vi "test_acquire_image.vi"() -> ()   [LabVIEW 2019, in "Picam.lvclass"]
uses:
  Picam.lvclass
  picam32_LabView_SDK/PICam_lib/types/PicamModel.ctl
  picam32_LabView_SDK/PICam_lib/types/PicamRoi.ctl
panel:
  in  "PicamRoi":T1={"x"=0, "width"=1024, "x_binning"=8, "y"=0, "height"=1024, "y_binning"=4}
  out "size(s)":i32[](array[numeric])
  out "ReadoutCount":i64
  out "Image":u16[][](graph)
  out "error out":errorcluster
  in  "PicamModel":T2=715 items=["---PIXIS 100 SERIES---"=1000, "PixisSeries"=0, "Pixis100BR"=5, "---PI-MAX4 SERIES---"=1001, "Pimax4Series"=700, "PiMax41024EM"=715]
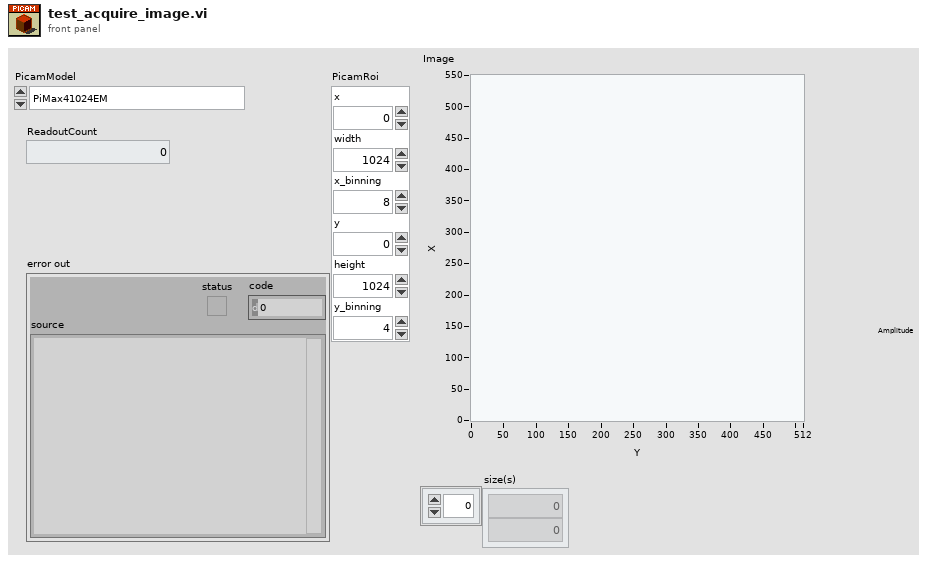
[diagram p1: front panel]
types:
  T1 = typedef "PicamRoi.ctl" = cluster{"x":i32, "width":i32, "x_binning":i32, "y":i32, "height":i32, "y_binning":i32}
  T2 = typedef "PicamModel.ctl" = u32
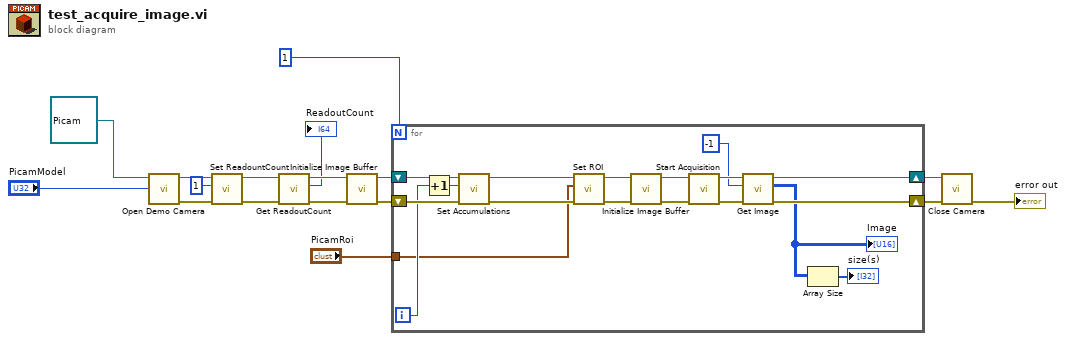
[diagram p0: block diagram]
diagram:
  n1 = call-dynamic "Open Demo Camera.vi"("PicamModel"="PicamModel", "Picam in"=refnum<class "Picam.lvclass"> refnum) -> ("error out"=w15:errorcluster, "Picam out"=w8:refnum<class "Picam.lvclass">)  [unwired: 8 in]
  n2 = call-dynamic "Set ReadountCount.vi"("error in (no error)"=w15, "ParameterValue"=i64 1, "Picam in"=w8) -> ("error out"=w9:errorcluster, "Picam out"=w5:refnum<class "Picam.lvclass">)  [unwired: 7 in]
  n3 = call-dynamic "Get ReadoutCount.vi"("error in (no error)"=w9, "Picam in"=w5) -> ("error out"=w6:errorcluster, "ParameterValue"=→"ReadoutCount":i64, "Picam out"=w4:refnum<class "Picam.lvclass">)  [unwired: 7 in]
  n4 = call-dynamic "Initialize Image Buffer.vi"("error in (no error)"=w6, "Picam in"=w4) -> ("error out"=w14:errorcluster, "Picam out"=w13:refnum<class "Picam.lvclass">)  [unwired: 8 in]
  n5 = for {
    N: 1 -> [_]
    shift-right: [w32] -> w12
    shift-left: w14 -> [w35]
    shift-right: [w31] -> w11
    shift-left: w13 -> [w26]
    tunnel: "PicamRoi" -> [w21]
    i -> [w25]
    n6 = Increment(x=w25) -> (x+1=w24:i32)
    n7 = call-dynamic "Set Accumulations.vi"("error in (no error)"=w35, "Accumulations"=w24, "Picam in"=w26) -> ("error out"=w27:errorcluster, "Picam out"=w22:refnum<class "Picam.lvclass">)  [unwired: 7 in]
    n8 = call-dynamic "Set ROI.vi"("error in (no error)"=w27, "PicamRoi"=w21, "Picam in"=w22) -> ("error out"=w23:errorcluster, "Picam out"=w19:refnum<class "Picam.lvclass">)  [unwired: 7 in]
    n9 = call-dynamic "Initialize Image Buffer.vi"("error in (no error)"=w23, "Picam in"=w19) -> ("error out"=w20:errorcluster, "Picam out"=w18:refnum<class "Picam.lvclass">)  [unwired: 8 in]
    n10 = call-dynamic "Start Acquisition.vi"("error in (no error)"=w20, "Picam in"=w18) -> ("error out"=w34:errorcluster, "Picam out"=w33:refnum<class "Picam.lvclass">)  [unwired: 8 in]
    n11 = call-dynamic "Get Image.vi"("error in (no error)"=w34, "Readout Timeout"=i64 -1, "Picam in"=w33) -> ("error out"=w32:errorcluster, "Image"=w29:u16[][], "Picam out"=w31:refnum<class "Picam.lvclass">)  [unwired: 6 in]
    "Image" <- w29
    n12 = Array Size(array=w29) -> (size(s)=→"size(s)":i32[])
  }
  n13 = call-dynamic "Close Camera.vi"("error in (no error)"=w12, "Picam in"=w11) -> ("error out"=→"error out":errorcluster)  [unwired: 8 in, 1 out]
